vi "W7X2DPut_DAZ.vi"(4 "dimensions":i64[](array[numeric])=[1399090569999999999, -1], 6 "pulse_length":dbl, 7 "Unit":string, 8 "sample period":dbl, 9 "sample rate":u16, 10 "SigJSONbuffer":string, 11 "SigLabel":string) -> (0 "Parlog error out":errorcluster)   [LabVIEW 2014]
uses:
  <vilib>/httpClient/POSTBuffer.vi
  <vilib>/httpClient/LabVIEWHTTPClient.lvlib
panel:
  out "JSON string":string
  in  "values":T1(array[cluster])=[{"sample_period"=0.004, "sample_rate"=2500, "pulse_length"=4.0, "detector"="Au_Kapton", "NChannels"=96, "ADCBits"=16, "chanDescs"=[{"name"="HBCm_U30_01", "active"=1, "physicalQuantity"={"type"="A"}}, {"name"="HBCm_U30_02", "active"=1, "physicalQuantity"={"type"="A"}}, {"name"="HBCm_U30_03", "active"=1, "physicalQuantity"={"type"="A"}}, {"name"="HBCm_U30_04", "active"=1, "physicalQuantity"={"type"="A"}}, {"name"="HBCm_U30_05", "active"=1, "physicalQuantity"={"type"="A"}}, {"name"="HBCm_U30_06", "active"=1, "physicalQuantity"={"type"="A"}}, {"name"="HBCm_U30_07", "active"=1, "physicalQuantity"={"type"="A"}}, {"name"="HBCm_U30_08", "active"=1, "physicalQuantity"={"type"="A"}}, {"name"="HBCm_U30_09", "active"=1, "physicalQuantity"={"type"="A"}}, {"name"="HBCm_U30_10", "active"=1, "physicalQuantity"={"type"="A"}}, {"name"="HBCm_U30_11", "active"=1, "physicalQuantity"={"type"="A"}}, {"name"="HBCm_U30_12", "active"=1, "physicalQuantity"={"type"="A"}}, {"name"="HBCm_U30_013", "active"=1, "physicalQuantity"={"type"="A"}}, {"name"="HBCm_U30_14", "active"=1, "physicalQuantity"={"type"="A"}}, {"name"="HBCm_U30_15", "active"=1, "physicalQuantity"={"type"="A"}}, {"name"="HBCm_U30_16", "active"=1, "physicalQuantity"={"type"="A"}}, {"name"="HBCm_U30_17", "active"=1, "physicalQuantity"={"type"="A"}}, {"name"="HBCm_U30_18", "active"=1, "physicalQuantity"={"type"="A"}}, {"name"="HBCm_U30_19", "active"=1, "physicalQuantity"={"type"="A"}}, {"name"="HBCm_U30_20", "active"=1, "physicalQuantity"={"type"="A"}}, {"name"="HBCm_U30_21", "active"=1, "physicalQuantity"={"type"="A"}}, {"name"="HBCm_U30_22", "active"=1, "physicalQuantity"={"type"="A"}}, {"name"="HBCm_U30_23", "active"=1, "physicalQuantity"={"type"="A"}}, {"name"="HBCm_U30_24", "active"=1, "physicalQuantity"={"type"="A"}}, {"name"="HBCm_U30_25", "active"=1, "physicalQuantity"={"type"="A"}}, {"name"="HBCm_U30_26", "active"=1, "physicalQuantity"={"type"="A"}}, {"name"="HBCm_U30_27", "active"=1, "physicalQuantity"={"type"="A"}}, {"name"="HBCm_U30_28", "active"=1, "physicalQuantity"={"type"="A"}}, {"name"="HBCm_U30_29", "active"=1, "physicalQuantity"={"type"="A"}}, {"name"="HBCm_U30_30", "active"=1, "physicalQuantity"={"type"="A"}}, {"name"="HBCm_U30_31", "active"=1, "physicalQuantity"={"type"="A"}}, {"name"="HBCm_U30_32", "active"=1, "physicalQuantity"={"type"="A"}}, {"name"="VBCm_V21_01", "active"=1, "physicalQuantity"={"type"="A"}}, {"name"="VBCm_V21_02", "active"=1, "physicalQuantity"={"type"="A"}}, {"name"="VBCm_V21_03", "active"=1, "physicalQuantity"={"type"="A"}}, {"name"="VBCm_V21_04", "active"=1, "physicalQuantity"={"type"="A"}}, {"name"="VBCm_V21_05", "active"=1, "physicalQuantity"={"type"="A"}}, {"name"="VBCm_V21_06", "active"=1, "physicalQuantity"={"type"="A"}}, {"name"="VBCm_V21_07", "active"=1, "physicalQuantity"={"type"="A"}}, {"name"="VBCm_V21_08", "active"=1, "physicalQuantity"={"type"="A"}}, {"name"="VBCm_V21_09", "active"=1, "physicalQuantity"={"type"="A"}}, {"name"="VBCm_V21_10", "active"=1, "physicalQuantity"={"type"="A"}}, {"name"="VBCm_V21_11", "active"=1, "physicalQuantity"={"type"="A"}}, {"name"="VBCm_V21_12", "active"=1, "physicalQuantity"={"type"="A"}}, {"name"="VBCm_V21_13", "active"=1, "physicalQuantity"={"type"="A"}}, {"name"="VBCm_V21_14", "active"=1, "physicalQuantity"={"type"="A"}}, {"name"="VBCm_V21_15", "active"=1, "physicalQuantity"={"type"="A"}}, {"name"="VBCm_V21_16", "active"=1, "physicalQuantity"={"type"="A"}}, {"name"="VBCm_V21_17", "active"=1, "physicalQuantity"={"type"="A"}}, {"name"="VBCm_V21_18", "active"=1, "physicalQuantity"={"type"="A"}}, {"name"="VBCm_V21_19", "active"=1, "physicalQuantity"={"type"="A"}}, {"name"="VBCm_V21_20", "active"=1, "physicalQuantity"={"type"="A"}}, {"name"="VBCm_V21_21", "active"=1, "physicalQuantity"={"type"="A"}}, {"name"="VBCm_V21_22", "active"=1, "physicalQuantity"={"type"="A"}}, {"name"="VBCm_V21_23", "active"=1, "physicalQuantity"={"type"="A"}}, {"name"="VBCm_V21_24", "active"=1, "physicalQuantity"={"type"="A"}}, {"name"="VBCm_V21_25", "active"=1, "physicalQuantity"={"type"="A"}}, {"name"="VBCm_V21_26", "active"=1, "physicalQuantity"={"type"="A"}}, {"name"="VBCm_V21_27", "active"=1, "physicalQuantity"={"type"="A"}}, {"name"="VBCm_V21_28", "active"=1, "physicalQuantity"={"type"="A"}}, {"name"="VBCm_V21_29", "active"=1, "physicalQuantity"={"type"="A"}}, {"name"="VBCm_V21_30", "active"=1, "physicalQuantity"={"type"="A"}}, {"name"="VBCm_V21_31", "active"=1, "physicalQuantity"={"type"="A"}}, {"name"="VBCm_V21_32", "active"=1, "physicalQuantity"={"type"="A"}}, {"name"="VBCm_V21_33", "active"=1, "physicalQuantity"={"type"="A"}}, {"name"="VBCm_V21_34", "active"=1, "physicalQuantity"={"type"="A"}}, {"name"="VBCm_V21_35", "active"=1, "physicalQuantity"={"type"="A"}}, {"name"="VBCm_V21_36", "active"=1, "physicalQuantity"={"type"="A"}}, {"name"="VBCm_V21_37", "active"=1, "physicalQuantity"={"type"="A"}}, {"name"="VBCm_V21_38", "active"=1, "physicalQuantity"={"type"="A"}}, {"name"="VBCm_V21_39", "active"=1, "physicalQuantity"={"type"="A"}}, {"name"="VBCm_V21_40", "active"=1, "physicalQuantity"={"type"="A"}}, {"name"="VBCs_V21_01", "active"=1, "physicalQuantity"={"type"="A"}}, {"name"="VBCs_V21_02", "active"=1, "physicalQuantity"={"type"="A"}}, {"name"="VBCs_V21_03", "active"=1, "physicalQuantity"={"type"="A"}}, {"name"="VBCs_V21_04", "active"=1, "physicalQuantity"={"type"="A"}}, {"name"="VBCs_V21_05", "active"=1, "physicalQuantity"={"type"="A"}}, {"name"="VBCs_V21_06", "active"=1, "physicalQuantity"={"type"="A"}}, {"name"="VBCs_V21_07", "active"=1, "physicalQuantity"={"type"="A"}}, {"name"="VBCs_V21_08", "active"=1, "physicalQuantity"={"type"="A"}}, {"name"="HBCs_U30_01", "active"=1, "physicalQuantity"={"type"="A"}}, {"name"="HBCs_U30_02", "active"=1, "physicalQuantity"={"type"="A"}}, {"name"="HBCs_U30_03", "active"=1, "physicalQuantity"={"type"="A"}}, {"name"="HBCs_U30_04", "active"=1, "physicalQuantity"={"type"="A"}}, {"name"="HBCs_U30_05", "active"=1, "physicalQuantity"={"type"="A"}}, {"name"="HBCs_U30_06", "active"=1, "physicalQuantity"={"type"="A"}}, {"name"="HBCs_U30_07", "active"=1, "physicalQuantity"={"type"="A"}}, {"name"="HBCs_U30_08", "active"=1, "physicalQuantity"={"type"="A"}}, {"name"="HBCs_U30_09", "active"=1, "physicalQuantity"={"type"="A"}}, {"name"="HBCs_U30_10", "active"=1, "physicalQuantity"={"type"="A"}}, {"name"="HBCs_U30_11", "active"=1, "physicalQuantity"={"type"="A"}}, {"name"="HBCs_U30_12", "active"=1, "physicalQuantity"={"type"="A"}}, {"name"="HBCs_U30_13", "active"=1, "physicalQuantity"={"type"="A"}}, {"name"="HBCs_U30_14", "active"=1, "physicalQuantity"={"type"="A"}}, {"name"="HBCs_U30_15", "active"=1, "physicalQuantity"={"type"="A"}}, {"name"="HBCs_U30_16", "active"=1, "physicalQuantity"={"type"="A"}}], "BridgeVoltage (V)"=5.0}]
  out "body":string
  out "headers":string
  out "body Parlog":string
  out "headers parms":string
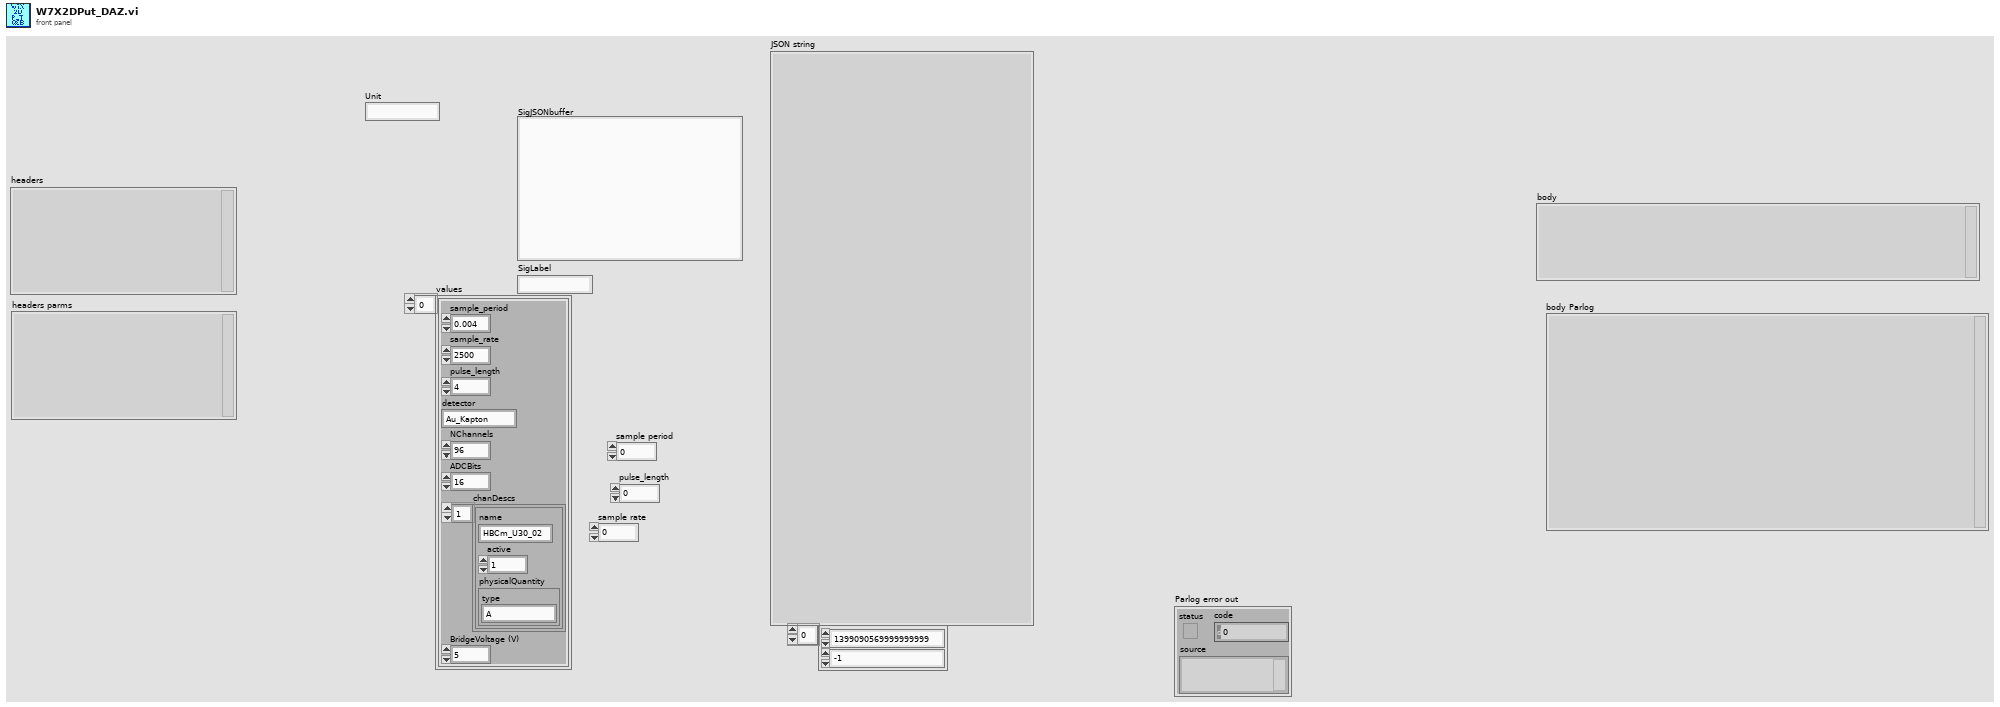
[diagram p1: front panel]
types:
  T1 = cluster{"sample_period":dbl, "sample_rate":u16, "pulse_length":dbl, "detector":string, "NChannels":u16, "ADCBits":u16, "chanDescs":cluster{"name":string, "active":i32, "physicalQuantity":cluster{"type":string}}[], "BridgeVoltage (V)":sgl}[]
  T2 = cluster{"sample_period":dbl, "sample_rate":u16, "pulse_length":dbl, "detector":string, "NChannels":u16, "ADCBits":u16, "chanDescs":cluster{"name":string, "active":i32, "physicalQuantity":cluster{"type":string}}[], "BridgeVoltage (V)":sgl}
  T3 = cluster{"name":string, "active":i32, "physicalQuantity":cluster{"type":string}}[]
  T4 = cluster{"name":string, "active":i32, "physicalQuantity":cluster{"type":string}}
  T5 = typedef "LabVIEWHTTPClient.lvlib/ClientHandle.ctl" = refnum<k1>
  T6 = cluster{"label":string, "values":cluster{"sample_period":dbl, "sample_rate":u16, "pulse_length":dbl, "detector":string, "NChannels":u16, "ADCBits":u16, "chanDescs":cluster{"name":string, "active":i32, "physicalQuantity":cluster{"type":string}}[], "BridgeVoltage (V)":sgl}[], "dimensions":i64[]}
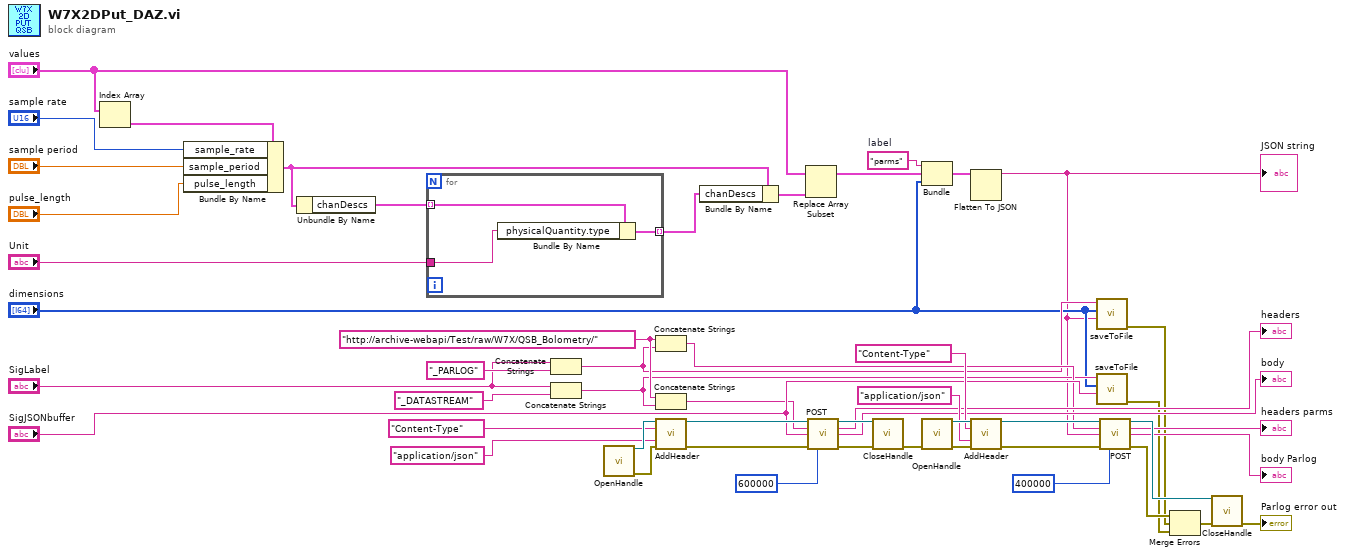
[diagram p0: block diagram]
diagram:
  w26 = "parms"  # label
  w9 = "http://archive-webapi/Test/raw/W7X/QSB_Bolometry/" ("url")
  n1 = Index Array(array="values") -> (element=w21:T2)  [unwired: 1 in]
  n2 = Bundle By Name(cluster=w21, "sample_rate"="sample rate", "sample_period"="sample period", "pulse_length"="pulse_length") -> (w17:T2)
  n3 = Unbundle By Name(w17) -> ("chanDescs"=w16:T3)
  n4 = for {
    tunnel: w16 -> [w54] mode=indexing
    tunnel: [w53] -> w15 mode=indexing
    tunnel: "Unit" -> [w52]
    n5 = Bundle By Name(cluster=w54, "physicalQuantity.type"=w52) -> (w53:T4)
  }
  n6 = Concatenate Strings("SigLabel", "_PARLOG" ("replace string (\"\")")) -> (w7:string)
  n7 = Concatenate Strings("SigLabel", "_DATASTREAM" ("string")) -> (w8:string)
  n8 = call <vilib>:"OpenHandle.vi"() -> ("client handle out"=w36:T5, "error out"=w35:errorcluster)  [unwired: 14 in]
  n9 = Concatenate Strings(w9, w7) -> (w10:string)
  n10 = Concatenate Strings(w9, w8) -> (w11:string)
  n11 = call <vilib>:"AddHeader.vi"("client handle"=w36, "header"="Content-Type", "value"="application/json", "error in (no error)"=w35) -> ("client handle out"=w34:T5, "error out"=w33:errorcluster)  [unwired: 10 in]
  n12 = Bundle By Name(cluster=w17, "chanDescs"=w15) -> (w19:T2)
  n13 = Replace Array Subset(array="values", new element=w19) -> (w18:T1)  [unwired: 1 in]
  n14 = call-poly <vilib>:"POST.vi"("client handle"=w34, "url"=w11, "buffer"="SigJSONbuffer", "error in (no error)"=w33, "timeout (10000)"=600000) -> ("client handle out"=w39:T5, "headers"=→"headers":string, "body"=→"body":string, "error out"=w38:errorcluster)  [unwired: 7 in]
  n15 = call <vilib>:"CloseHandle.vi"("client handle"=w39, "error in (no error)"=w38) -> ("error out"=w1:errorcluster)  [unwired: 13 in]
  n16 = Bundle("label"=w26, "values"=w18, "dimensions"="dimensions") -> (w25:T6)  [unwired: 1 in]
  n17 = call <vilib>:"OpenHandle.vi"("error in (no error)"=w1) -> ("client handle out"=w48:T5, "error out"=w47:errorcluster)  [unwired: 13 in]
  n18 = Flatten To JSON(anything=w25) -> (JSON string=w5:string)  [unwired: 2 in, 1 out]
  "JSON string" <- w5
  n19 = call <vilib>:"AddHeader.vi"("client handle"=w48, "header"="Content-Type", "value"="application/json", "error in (no error)"=w47) -> ("client handle out"=w46:T5, "error out"=w45:errorcluster)  [unwired: 10 in]
  n20 = call "saveToFile.vi"("SigJSONbuffer"=w5, "dimensions"="dimensions", "String"=w7) -> ("error out"=w3:errorcluster)  [unwired: 8 in]
  n21 = call "saveToFile.vi"("SigJSONbuffer"="SigJSONbuffer", "dimensions"="dimensions", "String"=w8) -> ("error out"=w2:errorcluster)  [unwired: 8 in]
  n22 = call-poly <vilib>:"POST.vi"("client handle"=w46, "url"=w10, "buffer"=w5, "error in (no error)"=w45, "timeout (10000)"=400000) -> ("client handle out"=w51:T5, "headers"=→"headers parms":string, "body"=→"body Parlog":string, "error out"=w50:errorcluster)  [unwired: 7 in]
  n23 = Merge Errors(w50, w3, w2) -> (w4:errorcluster)
  n24 = call <vilib>:"CloseHandle.vi"("client handle"=w51, "error in (no error)"=w4) -> ("error out"=→"Parlog error out":errorcluster)  [unwired: 13 in]
